vi "Test Open Message Handler Where Message Received.vi"(8 "error in (no error)":errorcluster, 11 "Test Case In":refnum<class "Debugger Test.lvclass">) -> (0 "error out":errorcluster, 3 "Test Case Out":refnum<class "Debugger Test.lvclass">)   [LabVIEW 2020, in "Debugger Test.lvclass"]
uses:
  Debugger Test.lvclass
  C:/Program Files (x86)/National Instruments/LabVIEW 2020/vi.lib/Astemes/LUnit/Test Case.lvclass
  source/Debugger/Debugger.lvclass
  C:/Users/anton/Documents/GitHub/triarc-debugger/source/Process/Debug Process.lvclass
  source/Debug Data/Raw Debug Data.ctl
  source/Process/Debug Process.lvclass/Debug Process.ctl
  <vilib>/Astemes/LUnit/Test Case.lvclass/Test Case.ctl
  <vilib>/Astemes/LUnit/LUnit Assertion Result.lvclass/LUnit Assertion Result.ctl
  <vilib>/Astemes/LUnit/LUnit Test Case Result.lvclass/LUnit Test Case Result.ctl
  <vilib>/Astemes/LUnit/LUnit Method Result.lvclass/LUnit Method Result.ctl
  01074fa8-ee8a-411d-bc8b-fc92c4f90959.vi
  source/Process/Private/SubVIs/Wait for finish.vi
  source/Process/Protected/Messaging/Enqueue Message.vi
  source/Process/Private/SubVIs/Set Lifecycle State.vi
  source/Process/Public/Lifecycle/Get Lifecycle State.vi
  <vilib>/Astemes/LUnit/Palette/Pass.vi
  <vilib>/Astemes/LUnit/Palette/Fail.vi
  <vilib>/Astemes/LUnit/Compare Variants.vi
  <vilib>/Astemes/LUnit/Describe Comparison.vi
  <vilib>/Astemes/LUnit/Set Assertion Type.vi
  <vilib>/Utility/error.llb/Clear Errors.vi
  <vilib>/Astemes/LUnit/Add test result.vi
  <vilib>/Astemes/LUnit/LUnit Write Passed.vi
  <vilib>/Astemes/LUnit/LUnit Write Message.vi
  <vilib>/Astemes/LUnit/LUnit Write Description.vi
  <vilib>/Astemes/LUnit/Variant to string.vi
  <vilib>/Astemes/LUnit/LUnit Write Assertion Type.vi
  <vilib>/Astemes/LUnit/LUnit Record Assertion Result.vi
  <vilib>/Astemes/LUnit/LUnit Aggregate Assertion Results.vi
  <vilib>/Astemes/LUnit/Assertion Result/LUnit Read Status.vi
  <vilib>/Astemes/LUnit/LUnit Read Message.vi
  <vilib>/Astemes/LUnit/LUnit Read Description.vi
  <vilib>/Astemes/LUnit/Method Result/LUnit Merge Status.vi
  <vilib>/Astemes/LUnit/LUnit Concatenate result strings.vi
  <vilib>/Utility/error.llb/Error Cluster From Error Code.vi
  <vilib>/Utility/Data Type/Get Type Information.vi
  <vilib>/Utility/LVClass/Get LV Class Name.vi
  <vilib>/Astemes/LUnit/LUnit Assertion Result.lvclass
  source/Process/Debug Process.lvclass
  Debugger Test.lvclass/Debugger Test.ctl
  source/Debug Data/Debug Data.lvclass
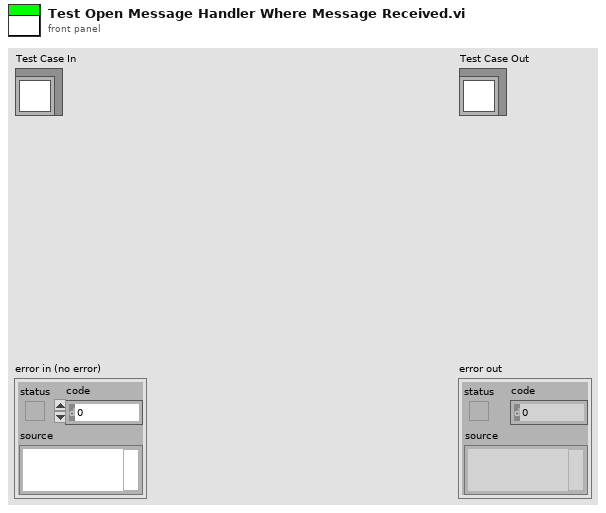
[diagram p1: front panel]
types:
  T1 = enum32{"Invalid", "Standard", "Closed", "Hidden", "Minimized", "Maximized"}
  T2 = typedef "Debug Data.lvclass/Raw Debug Data.ctl" = cluster{"Action":string, "Call Chain":string, "Process":string, "Message":string, "Message Data":variant, "Time":dbl}
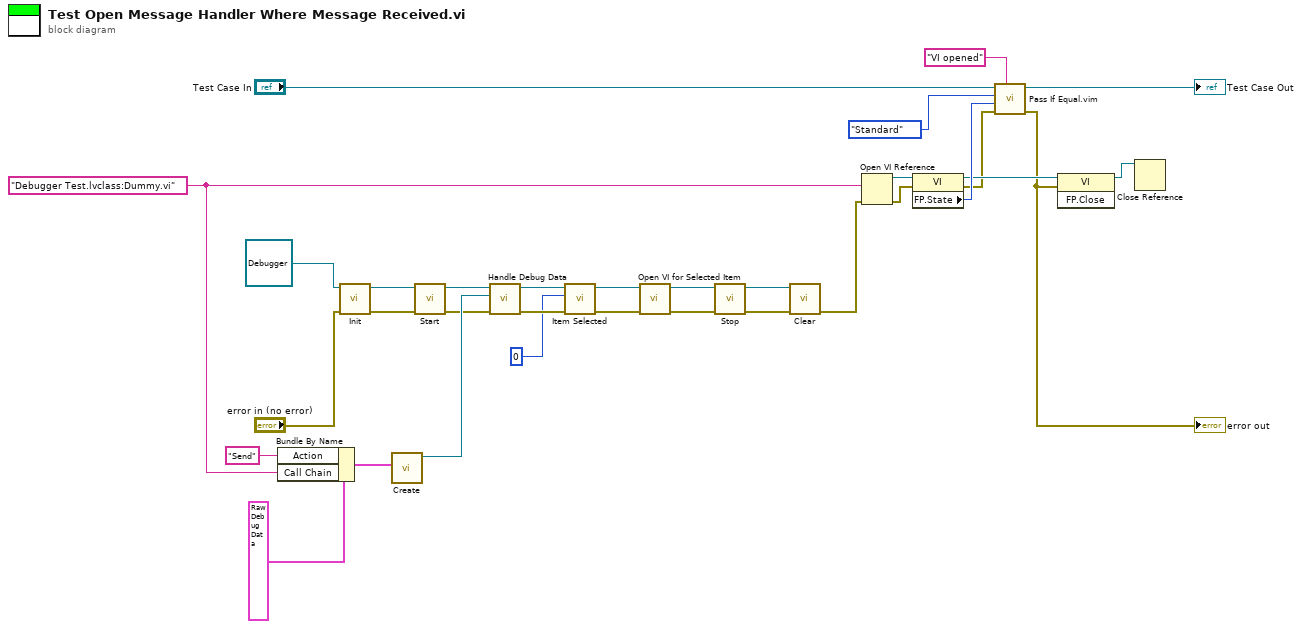
[diagram p0: block diagram]
diagram:
  w1 = "Debugger Test.lvclass:Dummy.vi"
  n1 = Bundle By Name(cluster=T2 {"Action"="", "Call Chain"="", "Process"="", "Message"="", "Message Data"=variant, "Time"=0.0} ("Debug Data Cluster"), "Action"="Send" ("Process"), "Call Chain"=w1) -> (w22:T2)
  n2 = call-dynamic "Init.vi"("error in (no error)"="error in (no error)", "Process In"=refnum<class "Debugger.lvclass"> refnum ("Debug Data Event In 2")) -> ("error out"=w29:errorcluster, "Process Out"=w30:refnum<class "Debugger.lvclass">)  [unwired: 8 in]
  n3 = call "Create.vi"("Debug Data Cluster"=w22) -> ("Debug Data out"=w23:refnum<class "Debug Data.lvclass">)  [unwired: 9 in, 1 out]
  n4 = call "Start.vi"("error in (no error)"=w29, "Process In"=w30) -> ("error out"=w18:errorcluster, "Process Out"=w19:refnum<class "Debugger.lvclass">)  [unwired: 7 in, 1 out]
  n5 = call-dynamic "Handle Debug Data.vi"("error in (no error)"=w18, "Debug Data.lvclass"=w23, "Debug Data Event In"=w19) -> ("error out"=w8:errorcluster, "Debug Data Event Out"=w9:refnum<class "Debugger.lvclass">)  [unwired: 7 in]
  n6 = call "Item Selected.vi"("error in (no error)"=w8, "Message ID"=u32 0, "Debugger in"=w9) -> ("error out"=w6:errorcluster, "Debugger out"=w7:refnum<class "Debugger.lvclass">)  [unwired: 7 in]
  n7 = call "Open VI for Selected Item.vi"("error in (no error)"=w6, "Debugger In"=w7) -> ("error out"=w4:errorcluster, "Debugger Out"=w5:refnum<class "Debugger.lvclass">)  [unwired: 8 in]
  n8 = call "Stop.vi"("error in (no error)"=w4, "Process In"=w5) -> ("error out"=w27:errorcluster, "Process Out"=w28:refnum<class "Debugger.lvclass">)  [unwired: 7 in, 1 out]
  n9 = call-dynamic "Clear.vi"("error in (no error)"=w27, "Process In"=w28) -> ("error out"=w10:errorcluster)  [unwired: 9 in]
  n10 = Open VI Reference(vi path=w1, error in (no error)=w10) -> (vi reference=w14:refnum<vi>, error out=w13:errorcluster)  [unwired: 4 in]
  n11 = property class="VI"(reference=w14, error in=w13) -> (reference out=w12:refnum<vi>, error out=w11:errorcluster, "FP.State"=w17:T1)
  n12 = call "Pass If Equal.vim"("Description"="VI opened", "error in (no error)"=w11, "Actual"=w17, "Expected"=T1."Standard" ("Front Panel Window:State"), "LUnit Test Case In"="Test Case In") -> ("error out"=w2:errorcluster, "LUnit Test Case Out"=→"Test Case Out":refnum<class "Debugger Test.lvclass">)  [unwired: 5 in]
  "error out" <- w2
  n13 = invoke class="VI" method="FP.Close"(reference=w12, error in=w2) -> (reference out=w15:refnum<vi>)  [unwired: 1 in, 2 out]
  n14 = Close Reference(reference=w15) -> ()  [unwired: 1 in, 1 out]
